vi "Settings.vi"(8 "error in (no error)":errorcluster, 9 "Gantry Region":i32=2, 11 "Component in":refnum<class "Component Tray.lvclass">) -> (0 "error out":errorcluster, 3 "Component out":refnum<class "Component Tray.lvclass">)   [LabVIEW 2016, in "Component Tray.lvclass"]
uses:
  Component Tray.lvclass
  D:/UCSB-Gantry/V5/Classes/Workspace/Fixture.lvclass
  Fixture.lvclass/Fixture.ctl
  Write Gantry Region.vi
  Write Fixture ID.vi
  Write Position.vi
panel:
  in  "6 Inch":bool
  in  "8 Inch":bool=TRUE
  in  "Position":i32=1
  in  "Tray Number":i32=2
  in  "Submit":bool
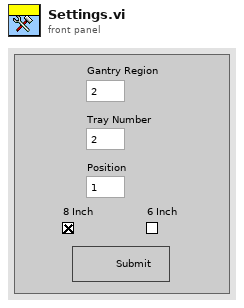
[diagram p1: front panel]
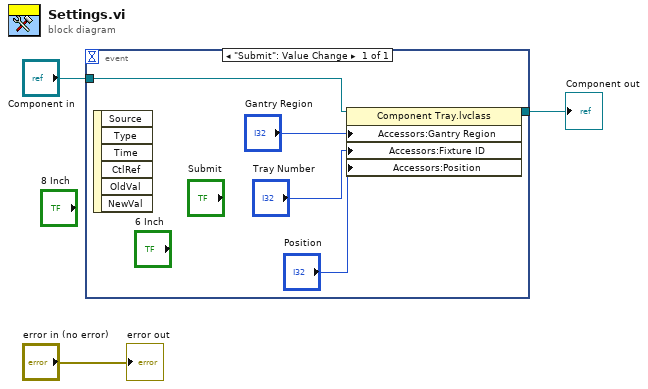
[diagram p0: block diagram]
diagram:
  n1 = event shown="[0] \"Submit\": Value Change" {
    selector: _ -> [_]
    dyn-events: _ -> [_]
    timeout: _ -> [_]
    tunnel: "Component in" -> [w8]
    tunnel: [w7] -> w1
    event "Submit": Value Change {
      n2 = event-data() -> ()  [unwired: 1 in, 6 out]
      n3 = property class="Component Tray.lvclass"(reference=w8, "Accessors:Gantry Region"="Gantry Region", "Accessors:Fixture ID"="Tray Number", "Accessors:Position"="Position") -> (reference out=w7:refnum<class "Component Tray.lvclass">)  [unwired: 1 in, 1 out]
    }
  }
  "Component out" <- w1
  "error out" <- "error in (no error)"
